vi "ghi_tc_poa_logger.vi"() -> ()   [LabVIEW 2021]
uses:
  <vilib>/ErrorRing/Error Ring.xnode
panel:
  out "Folder path":path
  in  "Stop measurement":bool
  out "Current timestamp":string
  out "Tin":dbl[](array[numeric])
  out "Temperatures":dynamicdata(graph)
  in  "Time (min)":dbl=1.0 caption="Delay Time (s)"
  out "T7":dbl[](array[numeric])
  out "T5":dbl[](array[numeric])
  out "T3":dbl[](array[numeric])
  out "T1":dbl[](array[numeric])
  out "error out":errorcluster
  out "Irradiance":dynamicdata(graph)
  in  "Thermocouple channels":string="1011,1013,1015,1017,1026"
  in  "RUN \nThermocouple":bool=TRUE
  in  "RUN \nirradiance 1030":bool=TRUE
  in  "RUN\nirradiance  1006":bool=TRUE
  out "Irradiance POA Front":dbl
  out "Irradiance POA Rear":dbl
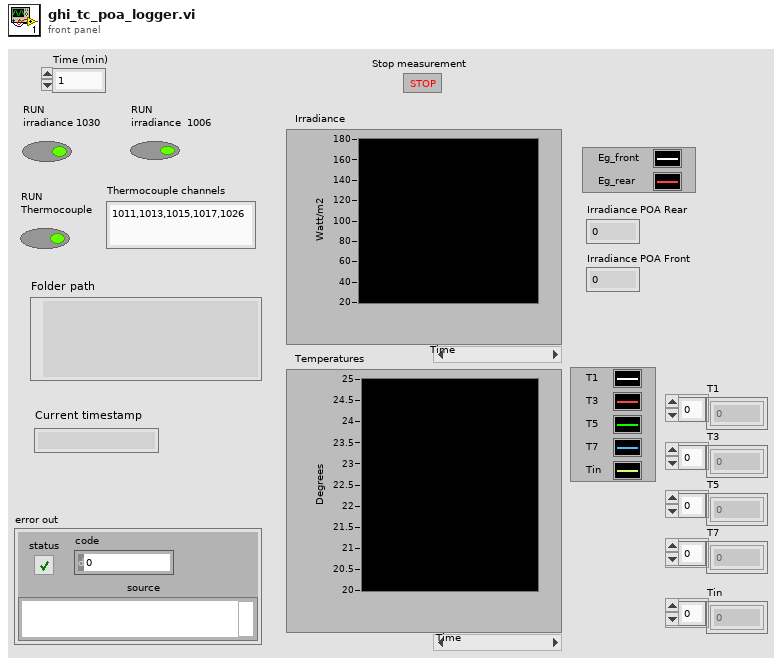
[diagram p1: front panel]
types:
  T1 = cluster{"Reference temperature[0]":dbl, "Reference temperature[1]":dbl, "Reference temperature[2]":dbl, "Reference temperature[3]":dbl, "Reference temperature[4]":dbl, "Reference temperature[5]":dbl, "Reference temperature[6]":dbl, "Reference temperature[7]":dbl, "Reference temperature[8]":dbl}
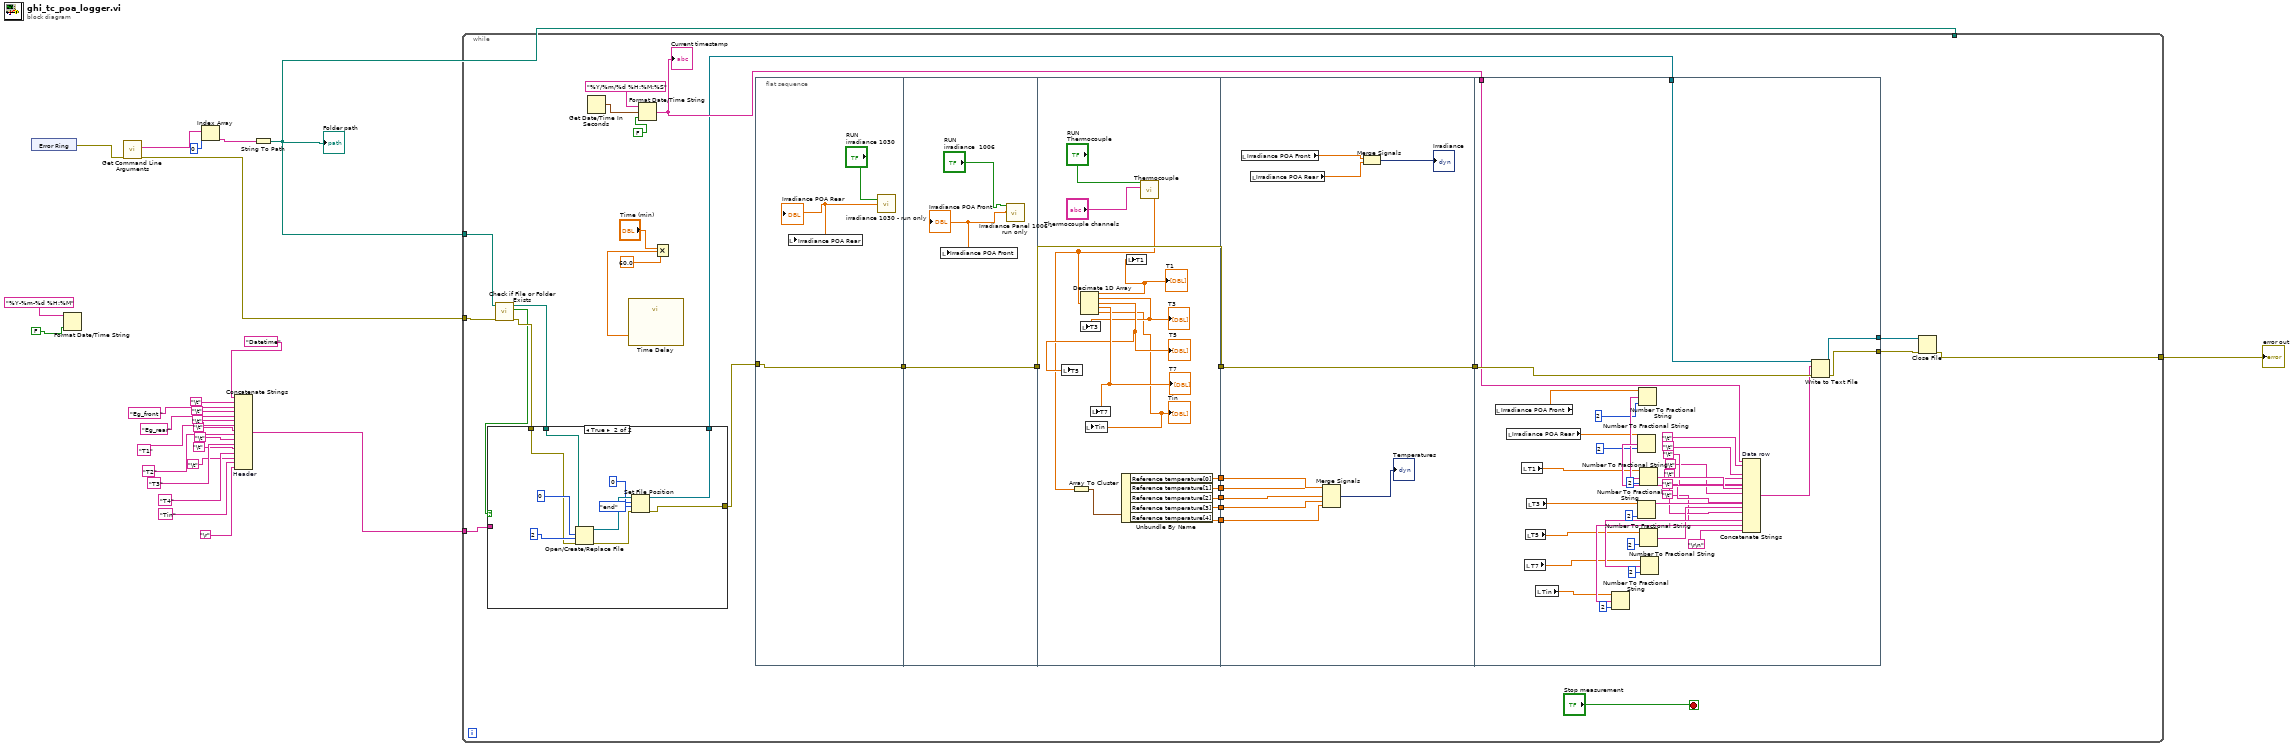
[diagram p0: block diagram]
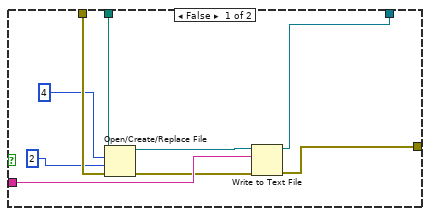
[diagram p2: hidden frame]
diagram:
  n1 = xnode "Error Ring"() -> ("error out"=w5:errorcluster)
  n2 = Format Date/Time String(time format string (%c)="%Y-%m-%d %H:%M", UTC format=FALSE ("want seconds? (F)")) -> ()  [unwired: 1 in, 1 out]
  n3 = call <vilib>:"Get Command Line Arguments.vi"("error in (no error)"=w5) -> ("error out"=w6:errorcluster, "arguments"=w3:string[])  [unwired: 8 in, 1 out]
  n4 = Index Array(array=w3, index=0) -> (element=w2:string)
  n5 = Concatenate Strings "Header"("Datetime" ("string"), "\t", "Eg_front " ("string"), "\t", "Eg_rear" ("string"), "\t", "T1" ("string"), "\t", "T2" ("string"), "\t", "T3" ("string"), "\t", "T4" ("string"), "\t", "Tin" ("string"), "\r") -> (w7:string)
  n6 = String To Path(string=w2) -> (path=w1:path)
  "Folder path" <- w1
  n7 = while "File Refnum\nLast close time" {
    tunnel: w1 -> [_]
    tunnel: [w35] -> w8
    tunnel: w7 -> [w34]
    tunnel: w6 -> [w31]
    tunnel: w1 -> [w30]
    stop <- "Stop measurement" stop-if-true
    n8 = call <vilib>:"Check if File or Folder Exists.vi"("error in (no error)"=w31, "path"=w30) -> ("error out"=w29:errorcluster, "file or folder exists?"=w28:bool, "dup path"=w27:path)  [unwired: 7 in]
    n9 = case shown="True" w28 {
      tunnel: w29 -> [w63 w71]
      tunnel: [w56 w65] -> w33
      tunnel: [w55 w68] -> w32
      tunnel: w27 -> [w62 w70]
      tunnel: w34 -> [w58 _]
      frame False {
        n10 = Open/Create/Replace File(file path (use dialog)=w62, error in=w63, operation (0:open)=4, access (0:read/write)=2) -> (refnum out=w59:refnum<file>, error out=w57:errorcluster)  [unwired: 2 in, 1 out]
        n11 = Write to Text File(file (use dialog)=w59, text=w58, error in=w57) -> (refnum out=w55:refnum<file>, error out=w56:errorcluster)  [unwired: 1 in, 1 out]
      }
      frame True {
        n12 = Open/Create/Replace File(file path (use dialog)=w70, error in=w71, operation (0:open)=0, access (0:read/write)=2) -> (refnum out=w69:refnum<file>, error out=w66:errorcluster)  [unwired: 2 in, 1 out]
        n13 = Set File Position(offset (in bytes) (0)=0, refnum=w69, from (0:start)=enum16{"start", "end", "current"}."end", error in=w66) -> (refnum out=w68:refnum<file>, error out=w65:errorcluster)
      }
    }
    n14 = Get Date/Time In Seconds() -> (seconds since 1Jan1904=w38:timestamp)
    n15 = Format Date/Time String(time format string (%c)="%Y/%m/%d %H:%M:%S", seconds (now)=w38, UTC format=FALSE ("want seconds? (F)")) -> (date/time string=w39:string)
    "Current timestamp" <- w39
    n16 = Multiply(x="Time (min)", y=60.0) -> (x*y=w50:dbl)
    n17 = call "Time Delay"("Delay Time (s)"=w50) -> ()  [unwired: 10 in, 1 out]
    n18 = flat-sequence {
      tunnel: w33 -> [w74]
      tunnel: [w74] -> w54
      tunnel: [w79] -> w53
      tunnel: w54 -> [w79]
      tunnel: [w92] -> w52
      tunnel: w53 -> [w92]
      tunnel: [w86] -> w47
      tunnel: [w85] -> w46
      tunnel: [w84] -> w45
      tunnel: [w83] -> w44
      tunnel: [w80] -> w43
      tunnel: [w101] -> w51
      tunnel: w52 -> [w101]
      tunnel: w47 -> [w99]
      tunnel: w46 -> [w98]
      tunnel: w45 -> [w97]
      tunnel: w44 -> [w96]
      tunnel: w43 -> [w95]
      tunnel: w51 -> [w139]
      tunnel: w39 -> [w108]
      tunnel: [w107] -> w37
      tunnel: [w106] -> w36
      tunnel: w32 -> [w105]
      frame #0 {
        n19 = call "irradiance 1030 - run only.vi"("Boolean"="RUN \nirradiance 1030") -> ("Irradiance"=w75:dbl)  [unwired: 10 in]
        "Irradiance POA Rear" <- w75
        n20 = local write "Irradiance POA Rear"(w75) -> ()
      }
      frame #1 {
        n21 = call "Irradiance Panel 1006 - run only.vi"("Boolean"="RUN\nirradiance  1006") -> ("Irradiance"=w77:dbl)  [unwired: 8 in]
        "Irradiance POA Front" <- w77
        n22 = local write "Irradiance POA Front"(w77) -> ()
      }
      frame #2 {
        n23 = call "Thermocouple.vi"("Thermocouple channels"="Thermocouple channels", "Start measure = True"="RUN \nThermocouple") -> ("Reference temperature"=w82:dbl[])  [unwired: 6 in]
        n24 = Array To Cluster(array=w82) -> (cluster=w87:T1)
        n25 = Decimate 1D Array(w82) -> (w88:dbl[], w89:dbl[], w90:dbl[], w91:dbl[], w81:dbl[])
        "T1" <- w88
        "T3" <- w89
        "T5" <- w90
        "T7" <- w91
        "Tin" <- w81
        n26 = local write "T5"(w90) -> ()
        n27 = local write "T3"(w89) -> ()
        n28 = local write "Tin"(w81) -> ()
        n29 = local write "T7"(w91) -> ()
        n30 = Unbundle By Name(w87) -> ("Reference temperature[0]"=w86:dbl, "Reference temperature[1]"=w85:dbl, "Reference temperature[2]"=w84:dbl, "Reference temperature[3]"=w83:dbl, "Reference temperature[4]"=w80:dbl)
        n31 = local write "T1"(w88) -> ()
      }
      frame #3 {
        n32 = local read "Irradiance POA Front"() -> (w104:dbl)
        n33 = local read "Irradiance POA Rear"() -> (w103:dbl)
        n34 = Merge Signals(w99, w98, w97, w96, w95) -> (→"Temperatures":dynamicdata)
        n35 = Merge Signals(w104, w103) -> (→"Irradiance":dynamicdata)
      }
      frame #4 {
        n36 = local read "Irradiance POA Front"() -> (w125:dbl)
        n37 = local read "Irradiance POA Rear"() -> (w126:dbl)
        n38 = local read "T1"() -> (w127:dbl[])
        n39 = local read "T7"() -> (w130:dbl[])
        n40 = local read "T5"() -> (w129:dbl[])
        n41 = local read "T3"() -> (w128:dbl[])
        n42 = local read "Tin"() -> (w137:dbl[])
        n43 = Number To Fractional String(number=w137, precision (6)=i16 2) -> (F-format string=w138:string[])  [unwired: 2 in]
        n44 = Number To Fractional String(number=w126, precision (6)=i16 2) -> (F-format string=w132:string)  [unwired: 2 in]
        n45 = Number To Fractional String(number=w128, precision (6)=i16 2) -> (F-format string=w134:string[])  [unwired: 2 in]
        n46 = Number To Fractional String(number=w125, precision (6)=2) -> (F-format string=w131:string)  [unwired: 2 in]
        n47 = Number To Fractional String(number=w127, precision (6)=i16 2) -> (F-format string=w133:string[])  [unwired: 2 in]
        n48 = Number To Fractional String(number=w129, precision (6)=i16 2) -> (F-format string=w135:string[])  [unwired: 2 in]
        n49 = Number To Fractional String(number=w130, precision (6)=i16 2) -> (F-format string=w136:string[])  [unwired: 2 in]
        n50 = Concatenate Strings "Data row"(w108, "\t", w131, "\t", w132, "\t", w133, "\t", w134, "\t", w135, "\t", w136, "\t", w138, "\r\n") -> (w109:string)
        n51 = Write to Text File(file (use dialog)=w105, text=w109, error in=w139) -> (refnum out=w106:refnum<file>, error out=w107:errorcluster)  [unwired: 1 in, 1 out]
      }
    }
    n52 = Close File(refnum=w36, error in=w37) -> (error out=w35:errorcluster)  [unwired: 1 out]
  }
  "error out" <- w8
